vi "여러신호시뮬레이션.vi"() -> ()   [LabVIEW 2014]
uses:
  <vilib>/measure/NI_MABase.lvlib
panel:
  in  "정지":bool
  in  "열거형":enum16{"사인파", "삼각파", "톱니파", "DC신호", "노이즈"}(ring)
  out "웨이브폼 그래프":waveform(dbl)(graph)
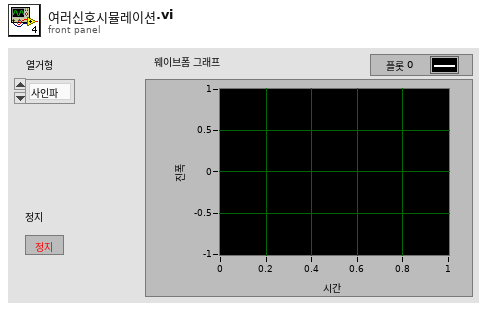
[diagram p1: front panel]
types:
  T1 = enum16{"Sine Wave", "Triangle Wave", "Square Wave", "Sawtooth Wave"}
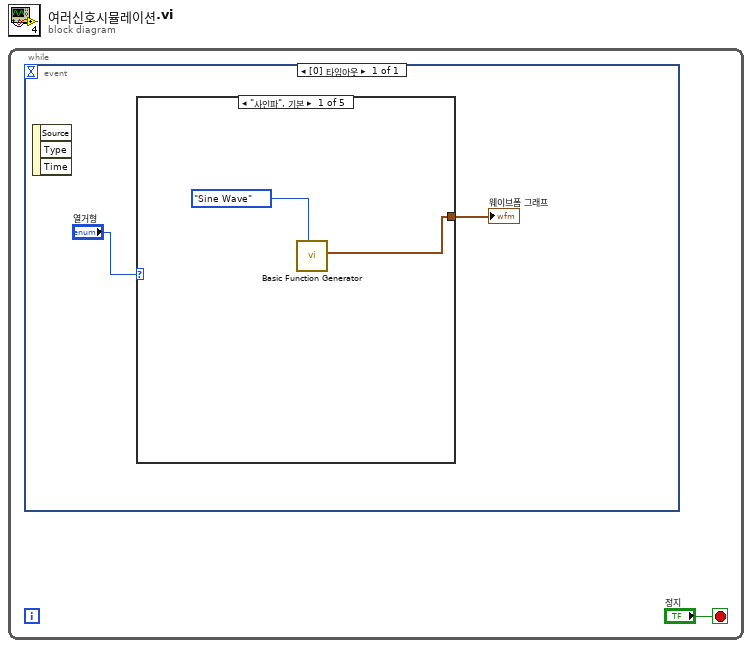
[diagram p0: block diagram]
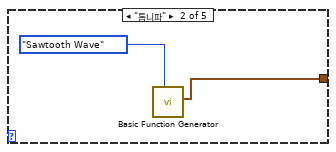
[diagram p2: hidden frame]
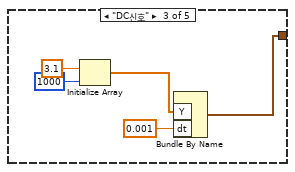
[diagram p3: hidden frame]
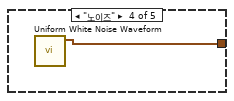
[diagram p4: hidden frame]
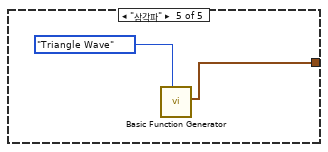
[diagram p5: hidden frame]
diagram:
  n1 = while {
    stop <- "정지" stop-if-true
    n2 = event shown="[0] 타임아웃" {
      selector: _ -> [_]
      dyn-events: _ -> [_]
      timeout: _ -> [_]
      event Timeout {
        n3 = event-data() -> ()  [unwired: 1 in, 3 out]
        n4 = case shown="\"사인파\", 기본" "열거형" {
          tunnel: [w4 w6 w8 w13 w15] -> w3
          frame "사인파", Default {
            n5 = call <vilib>:"Basic Function Generator.vi"("signal type"=T1."Sine Wave") -> ("signal out"=w4:waveform(dbl))  [unwired: 8 in, 2 out]
          }
          frame "톱니파" {
            n6 = call <vilib>:"Basic Function Generator.vi"("signal type"=T1."Sawtooth Wave") -> ("signal out"=w6:waveform(dbl))  [unwired: 8 in, 2 out]
          }
          frame "DC신호" {
            n7 = Initialize Array(3.1 ("원소"), 1000 ("차원 크기")) -> (w10:dbl[])
            n8 = Bundle By Name("Y"=w10, "dt"=0.001) -> (w8:waveform(dbl))  [unwired: 1 in]
          }
          frame "노이즈" {
            n9 = call <vilib>:"Uniform White Noise Waveform.vi"() -> ("signal out"=w13:waveform(dbl))  [unwired: 10 in, 1 out]
          }
          frame "삼각파" {
            n10 = call <vilib>:"Basic Function Generator.vi"("signal type"=T1."Triangle Wave") -> ("signal out"=w15:waveform(dbl))  [unwired: 8 in, 2 out]
          }
        }
        "웨이브폼 그래프" <- w3
      }
    }
  }
